vi "get_process_queue.vi"(8 "error in (no error)":errorcluster, 10 "Process name":string, 11 "Process_communication in":variant) -> (0 "error out":errorcluster, 1 "Process_control_queue":refnum<queue>, 3 "Process_communication out":variant)   [LabVIEW 2011, in "Fiberscope_library.lvlib"]
uses:
  Fiberscope_library.lvlib
  typedefs/control_process_state_cluster.ctl
  typedefs/control_process_state_enum.ctl
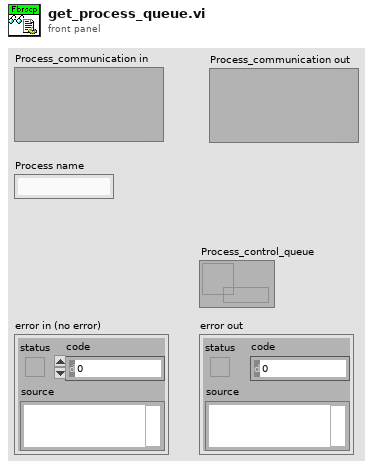
[diagram p1: front panel]
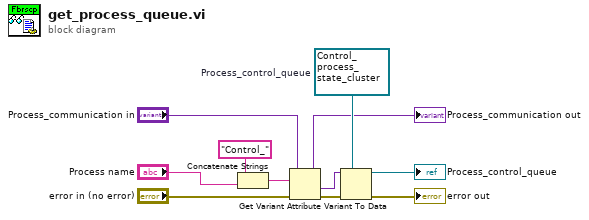
[diagram p0: block diagram]
diagram:
  w10 = refnum<queue> refnum  # Process_control_queue
  n1 = Concatenate Strings("Control_" ("string"), "Process name") -> (w6:string)
  n2 = Get Variant Attribute(Variant="Process_communication in", name=w6, error in="error in (no error)") -> (duplicate Variant=→"Process_communication out":variant, value=w9:variant, error out=w8:errorcluster)  [unwired: 1 in, 1 out]
  n3 = Variant To Data(error in=w8, type=w10, Variant=w9) -> (data=→"Process_control_queue":refnum<queue>, error out=→"error out":errorcluster)
